vi "Initialize Read From VS Engine.vi"(7 "Name":string, 8 "error in (no error)":errorcluster, 9 "FIFO Name":string, 10 "Refs":T4[](array[typedef]) format="%.0x", 11 "Item Ref in":T4 format="%.0x") -> (0 "error out":errorcluster, 2 "Read from VS Engine":T1 {"Pairs"."Refs"."Data Reference" format="%.0x"}, 3 "Device Ref out":T4 format="%.0x")   [LabVIEW 2015, in "Diagnostics Addon Engine.lvlib" / "Inline Async API.lvlib"]
uses:
  Inline Async API.lvlib
  <vilib>/NI Veristand/Custom Device API/Custom Device Item Ref.ctl
  Controls/Read From VS Engine.ctl
  <vilib>/NI Veristand/Custom Device API/Block Data Reference.ctl
  <vilib>/NI Veristand/Custom Device API/Data Reference.ctl
  <vilib>/NI Veristand/Custom Device API/Data Access Type.ctl
  <vilib>/NI Veristand/Custom Device API/Custom Device API.lvlib
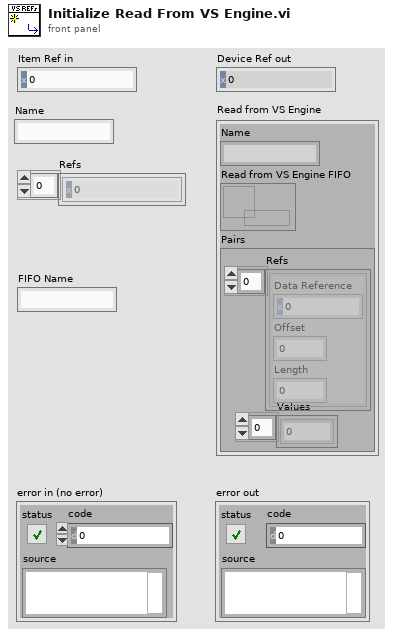
[diagram p1: front panel]
types:
  T1 = typedef "Diagnostics Addon Engine.lvlib/Inline Async API.lvlib/Read From VS Engine.ctl" = cluster{"Name":string, "Read from VS Engine FIFO":refnum<k33>, "Pairs":cluster{"Refs":T2[], "Values":dbl[]}}
  T2 = typedef "Custom Device API.lvlib/Block Data Reference.ctl" = cluster{"Data Reference":T3, "Offset":u64, "Length":u64}
  T3 = typedef "Custom Device API.lvlib/Data Reference.ctl" = i32
  T4 = typedef "Custom Device API.lvlib/Custom Device Item Ref.ctl" = u64
  T5 = typedef "Custom Device API.lvlib/Data Access Type.ctl" = enum16{"Read", "Write"}
  T6 = cluster{"read mode":enum16{"polling", "blocking"}, "write mode":enum16{"polling", "blocking"}}
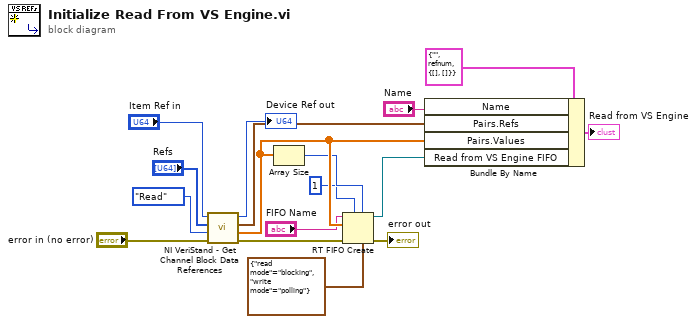
[diagram p0: block diagram]
diagram:
  n1 = call <vilib>:"NI VeriStand - Get Channel Block Data References.vi"("error in (no error)"="error in (no error)", "Access"=Data_Access_Type."Read", "Channel Refs"="Refs", "Device Ref in"="Item Ref in") -> ("error out"=w12:errorcluster, "Values Array"=w15:dbl[], "Block Data Refs"=w14:T2[], "Device Ref out"=→"Device Ref out":T4)  [unwired: 4 in]
  n2 = Array Size(array=w15) -> (size(s)=w5:i32)
  n3 = RT FIFO Create(0:"FIFO Name", 1:w15, 3:w12, 4:u32 1 ("size (10)"), 6:w5, 7:T6 {"read mode"=enum."blocking", "write mode"=enum."polling"} ("r/w modes (polling,polling)")) -> (8:w9:refnum<k33>, 11:→"error out":errorcluster)  [unwired: 2 in, 1 out]
  n4 = Bundle By Name(cluster=T1 {"Name"="", "Read from VS Engine FIFO"=refnum, "Pairs"={"Refs"=[], "Values"=[]}} ("Read from VS Engine"), "Name"="Name", "Pairs.Refs"=w14, "Pairs.Values"=w15, "Read from VS Engine FIFO"=w9) -> (→"Read from VS Engine":T1)
